vi "SUB_READ_COM1_Find2String_timeout.vi"(0 "duplicate VISA resource name 2":refnum<visa-resource-name>, 1 "Begin time":dbl, 2 "Timeout Seccond":dbl, 3 "Find String1":string, 4 "Find String2":string) -> (5 "Found String":bool, 6 "Output String":string, 7 "spent seconds":dbl)   [LabVIEW 2011]
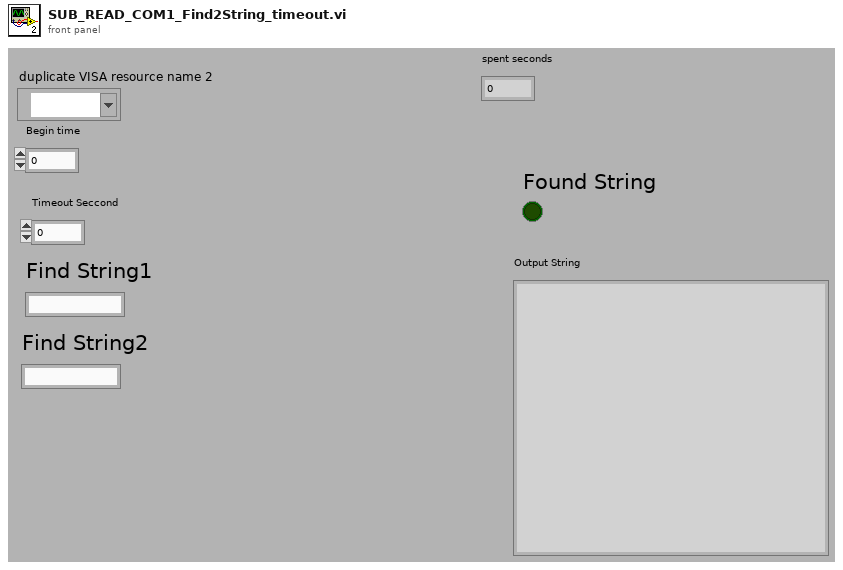
[diagram p1: front panel]
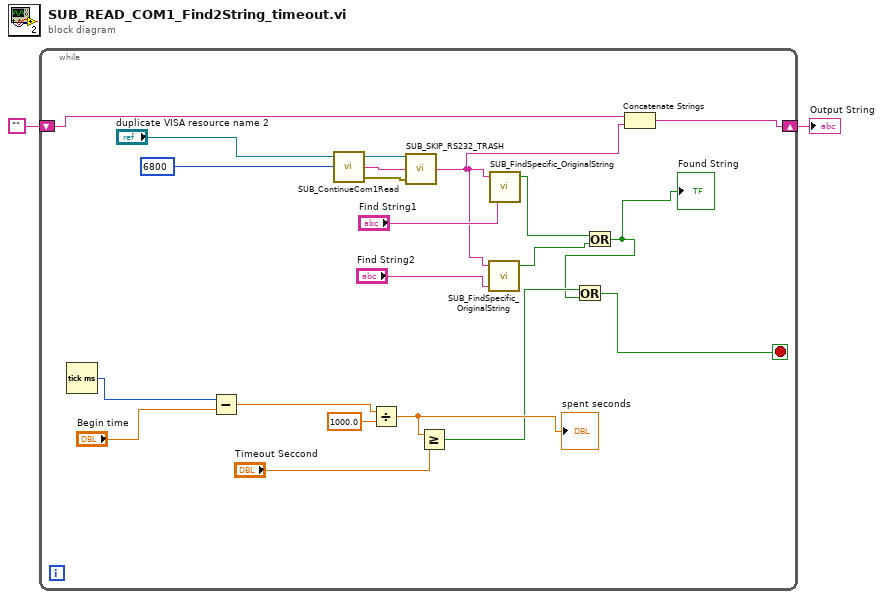
[diagram p0: block diagram]
diagram:
  n1 = while {
    shift-right: [w12] -> w1
    shift-left: "" -> [w11]
    stop <- w4 stop-if-true
    n2 = Tick Count (ms)() -> (millisecond timer value=w10:u32)
    n3 = Subtract(x=w10, y="Begin time") -> (x-y=w18:dbl)
    n4 = call "SUB_ContinueCom1Read.vi"("Numeric"=6800, "duplicate VISA resource name 2"="duplicate VISA resource name 2") -> ("error out"=w21:errorcluster, "String"=w22:string, "duplicate VISA resource name"=w23:refnum<visa-resource-name>)  [unwired: 1 in]
    n5 = Divide(x=w18, y=1000.0) -> (x/y=w16:dbl)
    "spent seconds" <- w16
    n6 = call "SUB_SKIP_RS232_TRASH.vi"("error out 2"=w21, "read buffer"=w22, "duplicate VISA resource name 2"=w23) -> ("String"=w7:string)  [unwired: 2 out]
    n7 = Greater Or Equal?(x=w16, y="Timeout Seccond") -> (x >= y?=w5:bool)
    n8 = call "SUB_FindSpecific_OriginalString.vi"("Find this String"="Find String2", "String data"=w7) -> ("Found"=w6:bool)  [unwired: 2 in, 1 out]
    n9 = call "SUB_FindSpecific_OriginalString.vi"("Find this String"="Find String1", "String data"=w7) -> ("Found"=w14:bool)  [unwired: 2 in, 1 out]
    n10 = Or(x=w14, y=w6) -> (x .or. y?=w3:bool)
    "Found String" <- w3
    n11 = Or(x=w5, y=w3) -> (x .or. y?=w4:bool)
    n12 = Concatenate Strings(w11, w7) -> (w12:string)
  }
  "Output String" <- w1
